vi "FRCts20_Backend_Processor.vi"() -> ()   [LabVIEW 2014, in "FRCts20_Backend_Engine.lvlib"]
doc: "The Processor VI represents the CPU for the Web Service system. All command messages are routed and handled by the central processor"
uses:
  FRCts20_Backend_Engine.lvlib
  FRCts20_Backend_FGVOperation.ctl
  FRCts20_Backend_DequeueDataOperations.ctl
  Dependencies/AMC/_SubVIs/TypeDefs/Message.ctl
  Dependencies/Keyed Array/KeyedArray.ctl
  <vilib>/addons/database/Connection.llb/DB Tools Open Connec (String).vi
  Dependencies/AMC/AMC.lvlib
  <vilib>/addons/database/NI_Database_API.lvlib
  INI_Accessor/FRCts20_Backend_INI Controller.lvclass
  Dependencies/Keyed Array/Tools_KeyedArray.lvlib
panel:
  out "Status":string
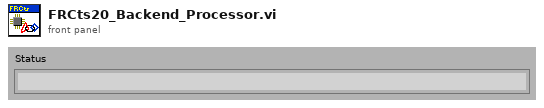
[diagram p1: front panel]
types:
  T1 = typedef "FRCts20_Backend_Engine.lvlib/FRCts20_Backend_EngineRefnums.ctl" = cluster{"Message Queue Methods":T2, "Message Queue Returns":T2, "Data Store Path":path, "Database Refnum":T3, "INI":refnum<class "FRCts20_Backend_INI Controller.lvclass">}
  T2 = typedef "AMC.lvlib/Message Queue.ctl" = refnum<queue>
  T3 = typedef "NI_Database_API.lvlib/Conn ObjectReference.ctl" = refnum<k1>
  T4 = typedef "FRCts20_Backend_Engine.lvlib/FRCts20_Backend_DequeueDataOperations.ctl" = enum16{"Initialize", "DequeueDataReturn", "GetQueues"}
  T5 = typedef "FRCts20_Backend_Engine.lvlib/FRCts20_Backend_FGVOperation.ctl" = enum16{"Initialize", "EnqueueMessage", "EnqueueDataReturn", "FlushMessage", "FlushDataReturn"}
  T6 = typedef "AMC.lvlib/Message.ctl" = cluster{"Name":string, "Value":string, "Attributes":T7, "Receiver Host":string, "Receiver Process":string, "Source Host":string, "Source Process":string, "Priority Message":bool, "Acknowledge Message":bool}
  T7 = typedef "Tools_KeyedArray.lvlib/KeyedArray.ctl" = cluster{"keys":string[], "values":string[]}
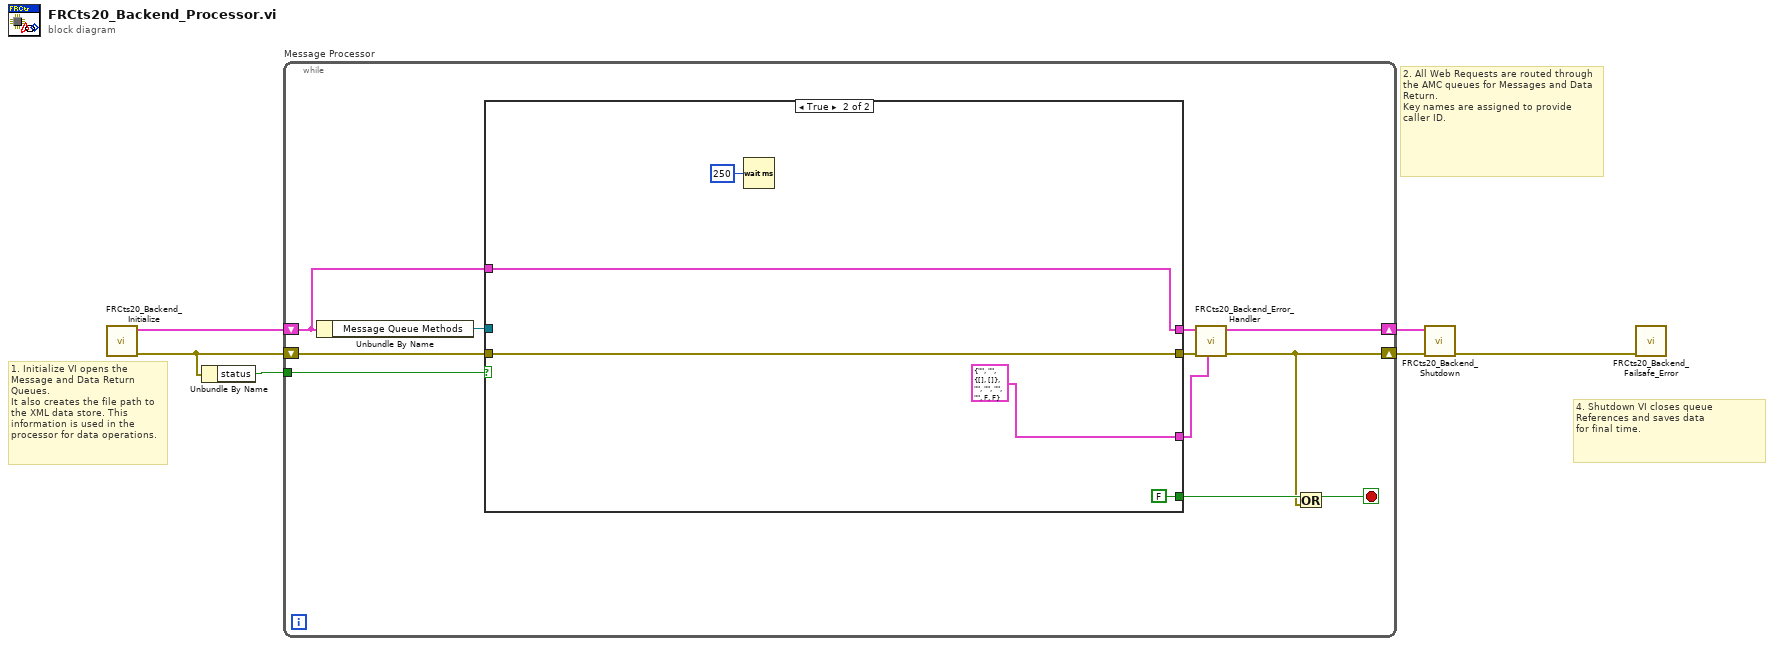
[diagram p0: block diagram]
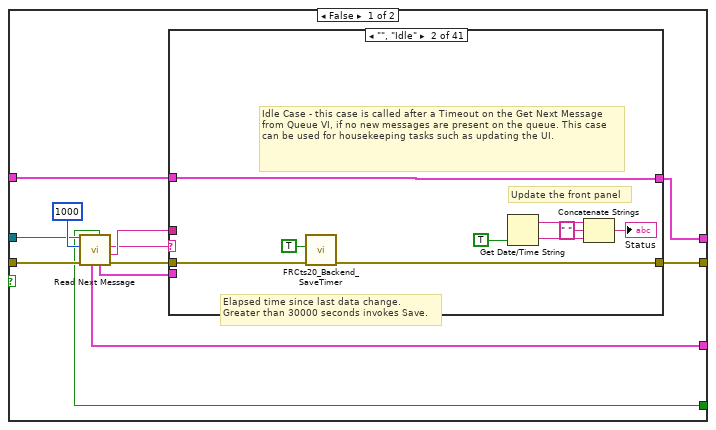
[diagram p2: hidden frame]
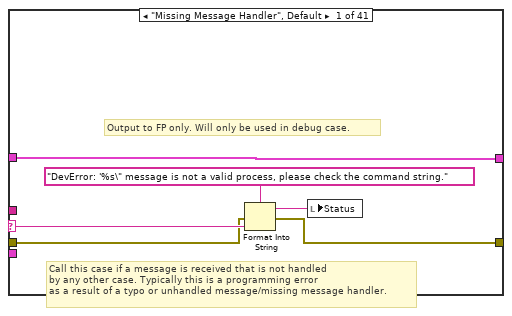
[diagram p3: hidden frame]
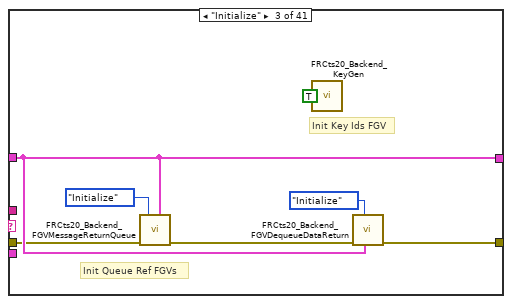
[diagram p4: hidden frame]
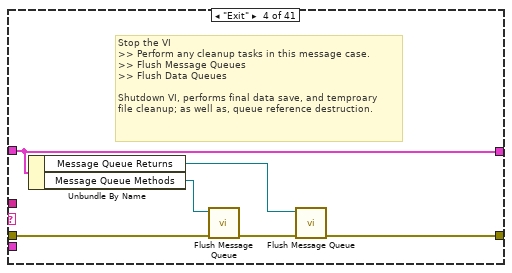
[diagram p5: hidden frame]
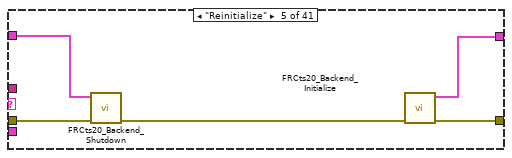
[diagram p6: hidden frame]
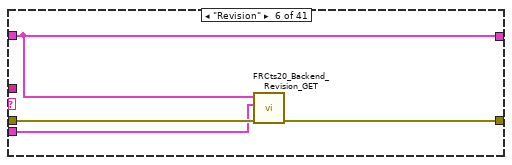
[diagram p7: hidden frame]
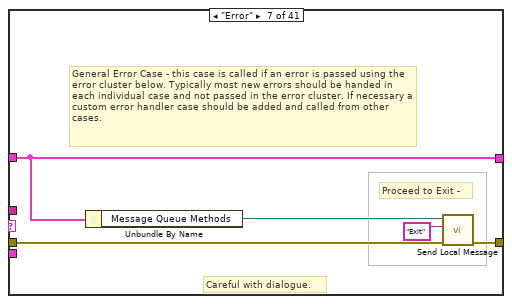
[diagram p8: hidden frame]
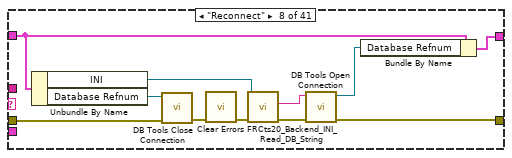
[diagram p9: hidden frame]
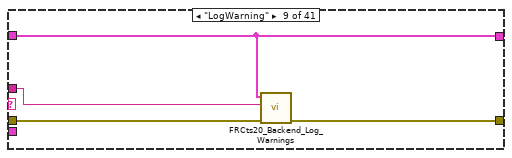
[diagram p10: hidden frame]
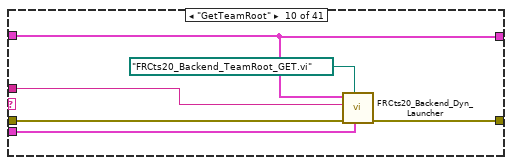
[diagram p11: hidden frame]
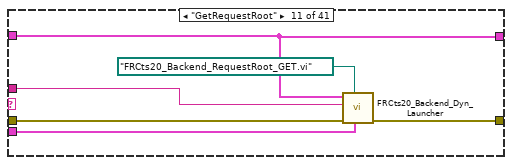
[diagram p12: hidden frame]
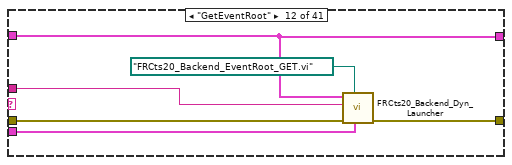
[diagram p13: hidden frame]
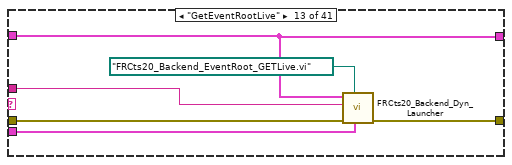
[diagram p14: hidden frame]
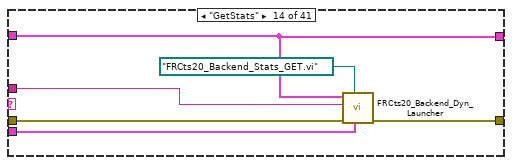
[diagram p15: hidden frame]
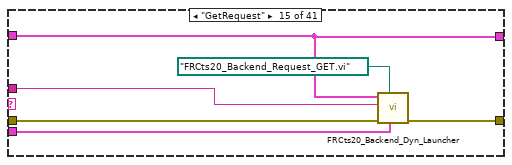
[diagram p16: hidden frame]
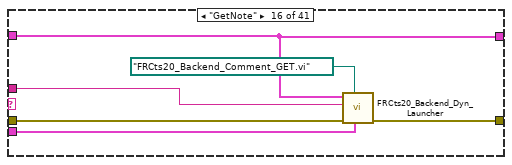
[diagram p17: hidden frame]
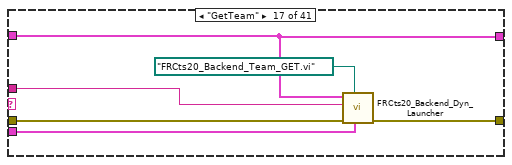
[diagram p18: hidden frame]
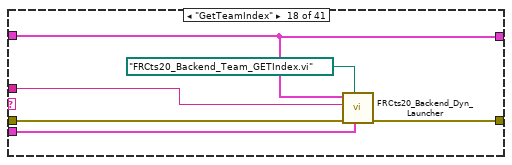
[diagram p19: hidden frame]
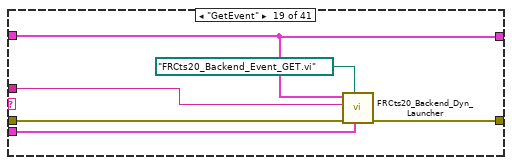
[diagram p20: hidden frame]
diagram:
  # "2. All Web Requests are routed through\nthe AMC queues for Messages and Data Return.\nKey names are assigned to provide caller ID."
  # "4. Shutdown VI closes queue References and saves data\nfor final time."
  # "1. Initialize VI opens the Message and Data Return Queues.\nIt also creates the file path to the XML data store. This \ninformation is used in the processor for data operations."
  n1 = call "FRCts20_Backend_Initialize.vi"() -> ("error out"=w2:errorcluster, "Engine_Refnums"=w5:T1)  [unwired: 10 in]
  n2 = Unbundle By Name(w2) -> ("status"=w1:bool)
  n3 = while "Message Processor" {
    shift-left: w2 -> [w10]
    shift-right: [w7] -> w6
    shift-right: [w12] -> w3
    shift-left: w5 -> [w16]
    tunnel: w1 -> [w11]
    stop <- w8 stop-if-true
    n4 = Unbundle By Name(w16) -> ("Message Queue Methods"=w17:T2)
    n5 = case shown="True" w11 {
      tunnel: w17 -> [w27 _]
      tunnel: w16 -> [w24 w290]
      tunnel: [w22 T6 {"Name"="", "Value"="", "Attributes"={"keys"=[], "values"=[]}, "Receiver Host"="", "Receiver Process"="", "Source Host"="", "Source Process"="", "Priority Message"=FALSE, "Acknowledge Message"=FALSE} ("Message")] -> w15
      tunnel: [w21 w288] -> w14
      tunnel: [w20 w290] -> w13
      tunnel: w10 -> [w19 w288]
      tunnel: [w18 FALSE ("Exit Process")] -> w9
      frame False {
        n6 = call "Read Next Message.vi"("error in (no error)"=w19, "timeout (1ms)"=1000 ("Timeout"), "Message Queue in"=w27) -> ("error out"=w29:errorcluster, "Message Value"=w26:string, "Message Name"=w23:string, "Message Attributes"=w25:T7, "Exit Process"=w18:bool, "Message"=w22:T6)  [unwired: 2 in, 1 out]
        n7 = case shown="\"\", \"Idle\"" w23 {
          selector: w23 -> [w35 _ _ _ _ _ _ _ _ _ _ _ _ _ _ _ _ _ _ _ _ _ _ _ _ _ _ _ _ _ _ _ _ _ _ _ _ _ _ _ _]
          tunnel: w29 -> [w31 w38 w46 w57 w61 w66 w68 w81 w85 w90 w96 w102 w108 w114 w120 w126 w132 w138 w144 w150 w156 w162 w168 w174 w180 w186 w192 w198 w204 w210 w216 w222 w228 w234 w240 w246 w252 w258 w264 w270 w277]
          tunnel: w26 -> [_ _ _ _ _ _ _ _ w83 w89 w95 w101 w107 w113 w119 w125 w131 w137 w143 w149 w155 w161 w167 w173 w179 w185 w191 w197 w203 w209 w215 w221 w227 w233 w239 w245 w251 w257 w263 w269 w276]
          tunnel: w25 -> [_ _ _ _ _ w63 _ _ _ w91 w97 w103 w109 w115 w121 w127 w133 w139 w145 w151 w157 w163 w169 w175 w181 w187 w193 w199 w205 w211 w217 w223 w229 w235 w241 w247 w253 w259 w265 w271 w278]
          tunnel: w24 -> [w33 w39 w47 w53 w60 w64 w67 w76 w86 w92 w98 w104 w110 w116 w122 w128 w134 w140 w146 w152 w158 w164 w170 w176 w182 w188 w194 w200 w206 w212 w218 w224 w230 w236 w242 w248 w254 w260 w266 w272 w273]
          tunnel: [w33 w39 w47 w53 w58 w64 w67 w77 w86 w92 w98 w104 w110 w116 w122 w128 w134 w140 w146 w152 w158 w164 w170 w176 w182 w188 w194 w200 w206 w212 w218 w224 w230 w236 w242 w248 w254 w260 w266 w272 w273] -> w20
          tunnel: [w30 w36 w45 w52 w59 w65 w69 w73 w84 w87 w93 w99 w105 w111 w117 w123 w129 w135 w141 w147 w153 w159 w165 w171 w177 w183 w189 w195 w201 w207 w213 w219 w225 w231 w237 w243 w249 w255 w261 w267 w274] -> w21
          frame "Missing Message Handler", Default {
            # "Output to FP only. Will only be used in debug case."
            # "Call this case if a message is received that is not handled \nby any other case. Typically this is a programming error\nas a result of a typo or unhandled message/missing message handler."
            n8 = Format Into String(format string="DevError: '%s\" message is not a valid process, please check the command string." ("message"), error in=w31, w35) -> (resulting string=w32:string, error out=w30:errorcluster)  [unwired: 1 in]
            n9 = local write "Status"(w32) -> ()
          }
          frame "", "Idle" {
            # "Elapsed time since last data change. \nGreater than 30000 seconds invokes Save."
            # "Update the front panel"
            # "Idle Case - this case is called after a Timeout on the Get Next Message from Queue VI, if no new messages are present on the queue. This case can be used for housekeeping tasks such as updating the UI."
            n10 = call "FRCts20_Backend_SaveTimer.vi"("error in (no error)"=w38, "Data Changed?"=TRUE) -> ("error out"=w36:errorcluster)  [unwired: 9 in]
            n11 = Get Date/Time String(want seconds? (F)=TRUE) -> (date string=w44:string, time string=w43:string)  [unwired: 2 out]
            n12 = Concatenate Strings(w44, " " ("string"), w43) -> (→"Status":string)
          }
          frame "Initialize" {
            # "Initialize competition start\ndate for stats generation"
            # "Init Queue Ref FGVs"
            # "Init Key Ids FGV"
            # "Primary Reference Initialization for Send/Return Queues"
            n13 = call "FRCts20_Backend_FGVMessageReturnQueue.vi"("Engine_Refnums"=w47, "Operation"=FRCts20_Backend_FGVOperation."Initialize", "error in (no error)"=w46) -> ("error out"=w50:errorcluster)  [unwired: 7 in, 1 out]
            n14 = call "FRCts20_Backend_KeyGen.vi"("Init?"=TRUE) -> ()  [unwired: 26 in, 1 out]
            n15 = call "FRCts20_Backend_FGVDequeueDataReturn.vi"("Engine_Refnums"=w47, "Operation"=FRCts20_Backend_DequeueDataOperations."Initialize", "error in (no error)"=w50) -> ("error out"=w45:errorcluster)  [unwired: 4 in, 4 out]
          }
          frame "Exit" {
            # "Stop the VI\n>> Perform any cleanup tasks in this message case.\n>> Flush Message Queues\n>> Flush Data Queues\n\nShutdown VI, performs final data save, and temproary\nfile cleanup; as well as, queue reference destruction."
            n16 = Unbundle By Name(w53) -> ("Message Queue Returns"=w54:T2, "Message Queue Methods"=w55:T2)
            n17 = call "Flush Message Queue.vi"("error in (no error)"=w57, "Message Queue in"=w55) -> ("error out"=w56:errorcluster)  [unwired: 7 in, 1 out]
            n18 = call "Flush Message Queue.vi"("error in (no error)"=w56, "Message Queue in"=w54) -> ("error out"=w52:errorcluster)  [unwired: 7 in, 1 out]
          }
          frame "Reinitialize" {
            n19 = call "FRCts20_Backend_Shutdown.vi"("error in (no error)"=w61, "Engine_Refnums"=w60) -> ("error out"=w62:errorcluster)  [unwired: 9 in]
            n20 = call "FRCts20_Backend_Initialize.vi"("error in (no error)"=w62) -> ("error out"=w59:errorcluster, "Engine_Refnums"=w58:T1)  [unwired: 9 in]
          }
          frame "Revision" {
            n21 = call "FRCts20_Backend_Revision_GET.vi"("error in (no error)"=w66, "Message Attributes"=w63, "Engine_Refnums"=w64) -> ("error out"=w65:errorcluster)  [unwired: 8 in]
          }
          frame "Error" {
            (unwired) errorcluster {"status"=FALSE, "code"=0, "source"=""} ("error out")
            # "Careful with dialogue."
            # "Proceed to Exit -"
            # "General Error Case - this case is called if an error is passed using the error cluster below. Typically most new errors should be handed in each individual case and not passed in the error cluster. If necessary a custom error handler case should be added and called from other cases."
            n22 = Unbundle By Name(w67) -> ("Message Queue Methods"=w70:T2)
            n23 = call "Send Local Message.vi"("error in (no error)"=w68, "Message Name"="Exit", "Message Queue in"=w70) -> ("error out"=w69:errorcluster)  [unwired: 3 in, 5 out]
          }
          frame "Reconnect" {
            n24 = Unbundle By Name(w76) -> ("INI"=w78:refnum<class "FRCts20_Backend_INI Controller.lvclass">, "Database Refnum"=w82:T3)
            n25 = call <vilib>:"DB Tools Close Connection.vi"("error in (no error)"=w81, "connection reference"=w82) -> ("error out"=w80:errorcluster)  [unwired: 5 in]
            n26 = call <vilib>:"Clear Errors.vi"("error in (no error)"=w80) -> ("error out"=w79:errorcluster)  [unwired: 5 in, 1 out]
            n27 = call "FRCts20_Backend_INI_Read_DB_String.vi"("error in (no error)"=w79, "INI Controller in"=w78) -> ("error out"=w74:errorcluster, "Connection String"=w75:string)  [unwired: 7 in, 1 out]
            n28 = call-poly <vilib>:"DB Tools Open Connection.vi"("error in (no error)"=w74, "connection information"=w75) -> ("error out"=w73:errorcluster, "connection reference"=w72:T3)  [unwired: 6 in]
            n29 = Bundle By Name(cluster=w76, "Database Refnum"=w72) -> (w77:T1)
          }
          frame "LogWarning" {
            n30 = call "FRCts20_Backend_Log_Warnings.vi"("error in (no error)"=w85, "Data"=w83, "Engine_Refnums"=w86) -> ("error out"=w84:errorcluster)  [unwired: 8 in]
          }
          frame "GetTeamRoot" {
            n31 = call "FRCts20_Backend_Dyn_Launcher.vi"("Message Attributes"=w91, "VI Name"=path "FRCts20_Backend_TeamRoot_GET.vi" ("VI Path"), "error in (no error)"=w90, "Data"=w89, "Engine_Refnums"=w92) -> ("error out"=w87:errorcluster)  [unwired: 6 in]
          }
          frame "GetRequestRoot" {
            n32 = call "FRCts20_Backend_Dyn_Launcher.vi"("Message Attributes"=w97, "VI Name"=path "FRCts20_Backend_RequestRoot_GET.vi" ("VI Path"), "error in (no error)"=w96, "Data"=w95, "Engine_Refnums"=w98) -> ("error out"=w93:errorcluster)  [unwired: 6 in]
          }
          frame "GetEventRoot" {
            n33 = call "FRCts20_Backend_Dyn_Launcher.vi"("Message Attributes"=w103, "VI Name"=path "FRCts20_Backend_EventRoot_GET.vi" ("VI Path"), "error in (no error)"=w102, "Data"=w101, "Engine_Refnums"=w104) -> ("error out"=w99:errorcluster)  [unwired: 6 in]
          }
          frame "GetEventRootLive" {
            n34 = call "FRCts20_Backend_Dyn_Launcher.vi"("Message Attributes"=w109, "VI Name"=path "FRCts20_Backend_EventRoot_GETLive.vi" ("VI Path"), "error in (no error)"=w108, "Data"=w107, "Engine_Refnums"=w110) -> ("error out"=w105:errorcluster)  [unwired: 6 in]
          }
          frame "GetStats" {
            n35 = call "FRCts20_Backend_Dyn_Launcher.vi"("Message Attributes"=w115, "VI Name"=path "FRCts20_Backend_Stats_GET.vi" ("VI Path"), "error in (no error)"=w114, "Data"=w113, "Engine_Refnums"=w116) -> ("error out"=w111:errorcluster)  [unwired: 6 in]
          }
          frame "GetRequest" {
            n36 = call "FRCts20_Backend_Dyn_Launcher.vi"("Message Attributes"=w121, "VI Name"=path "FRCts20_Backend_Request_GET.vi" ("VI Path"), "error in (no error)"=w120, "Data"=w119, "Engine_Refnums"=w122) -> ("error out"=w117:errorcluster)  [unwired: 6 in]
          }
          frame "GetNote" {
            n37 = call "FRCts20_Backend_Dyn_Launcher.vi"("Message Attributes"=w127, "VI Name"=path "FRCts20_Backend_Comment_GET.vi" ("VI Path"), "error in (no error)"=w126, "Data"=w125, "Engine_Refnums"=w128) -> ("error out"=w123:errorcluster)  [unwired: 6 in]
          }
          frame "GetTeam" {
            n38 = call "FRCts20_Backend_Dyn_Launcher.vi"("Message Attributes"=w133, "VI Name"=path "FRCts20_Backend_Team_GET.vi" ("VI Path"), "error in (no error)"=w132, "Data"=w131, "Engine_Refnums"=w134) -> ("error out"=w129:errorcluster)  [unwired: 6 in]
          }
          frame "GetTeamIndex" {
            n39 = call "FRCts20_Backend_Dyn_Launcher.vi"("Message Attributes"=w139, "VI Name"=path "FRCts20_Backend_Team_GETIndex.vi" ("VI Path"), "error in (no error)"=w138, "Data"=w137, "Engine_Refnums"=w140) -> ("error out"=w135:errorcluster)  [unwired: 6 in]
          }
          frame "GetEvent" {
            n40 = call "FRCts20_Backend_Dyn_Launcher.vi"("Message Attributes"=w145, "VI Name"=path "FRCts20_Backend_Event_GET.vi" ("VI Path"), "error in (no error)"=w144, "Data"=w143, "Engine_Refnums"=w146) -> ("error out"=w141:errorcluster)  [unwired: 6 in]
          }
          frame "GetEventFiltered" {
            n41 = call "FRCts20_Backend_Dyn_Launcher.vi"("Message Attributes"=w151, "VI Name"=path "FRCts20_Backend_Event_GETFiltered.vi" ("VI Path"), "error in (no error)"=w150, "Data"=w149, "Engine_Refnums"=w152) -> ("error out"=w147:errorcluster)  [unwired: 6 in]
          }
          frame "GetDivision" {
            n42 = call "FRCts20_Backend_Dyn_Launcher.vi"("Message Attributes"=w157, "VI Name"=path "FRCts20_Backend_Division_GET.vi" ("VI Path"), "error in (no error)"=w156, "Data"=w155, "Engine_Refnums"=w158) -> ("error out"=w153:errorcluster)  [unwired: 6 in]
          }
          frame "PostRequestRoot" {
            n43 = call "FRCts20_Backend_Dyn_Launcher.vi"("Message Attributes"=w163, "VI Name"=path "FRCts20_Backend_RequestRoot_POST.vi" ("VI Path"), "error in (no error)"=w162, "Data"=w161, "Engine_Refnums"=w164) -> ("error out"=w159:errorcluster)  [unwired: 6 in]
          }
          frame "PostNote" {
            n44 = call "FRCts20_Backend_Dyn_Launcher.vi"("Message Attributes"=w169, "VI Name"=path "FRCts20_Backend_Comment_POST.vi" ("VI Path"), "error in (no error)"=w168, "Data"=w167, "Engine_Refnums"=w170) -> ("error out"=w165:errorcluster)  [unwired: 6 in]
          }
          frame "PostEventRoot" {
            n45 = call "FRCts20_Backend_Dyn_Launcher.vi"("Message Attributes"=w175, "VI Name"=path "FRCts20_Backend_EventRoot_POST.vi" ("VI Path"), "error in (no error)"=w174, "Data"=w173, "Engine_Refnums"=w176) -> ("error out"=w171:errorcluster)  [unwired: 6 in]
          }
          frame "PostDivision" {
            n46 = call "FRCts20_Backend_Dyn_Launcher.vi"("Message Attributes"=w181, "VI Name"=path "FRCts20_Backend_Division_POST.vi" ("VI Path"), "error in (no error)"=w180, "Data"=w179, "Engine_Refnums"=w182) -> ("error out"=w177:errorcluster)  [unwired: 6 in]
          }
          frame "PostTeamRoot" {
            n47 = call "FRCts20_Backend_Dyn_Launcher.vi"("Message Attributes"=w187, "VI Name"=path "FRCts20_Backend_TeamRoot_POST.vi" ("VI Path"), "error in (no error)"=w186, "Data"=w185, "Engine_Refnums"=w188) -> ("error out"=w183:errorcluster)  [unwired: 6 in]
          }
          frame "PutRequest" {
            n48 = call "FRCts20_Backend_Dyn_Launcher.vi"("Message Attributes"=w193, "VI Name"=path "FRCts20_Backend_Request_PUT.vi" ("VI Path"), "error in (no error)"=w192, "Data"=w191, "Engine_Refnums"=w194) -> ("error out"=w189:errorcluster)  [unwired: 6 in]
          }
          frame "PutEvent" {
            n49 = call "FRCts20_Backend_Dyn_Launcher.vi"("Message Attributes"=w199, "VI Name"=path "FRCts20_Backend_Event_PUT.vi" ("VI Path"), "error in (no error)"=w198, "Data"=w197, "Engine_Refnums"=w200) -> ("error out"=w195:errorcluster)  [unwired: 6 in]
          }
          frame "PutDivision" {
            n50 = call "FRCts20_Backend_Dyn_Launcher.vi"("Message Attributes"=w205, "VI Name"=path "FRCts20_Backend_Division_PUT.vi" ("VI Path"), "error in (no error)"=w204, "Data"=w203, "Engine_Refnums"=w206) -> ("error out"=w201:errorcluster)  [unwired: 6 in]
          }
          frame "PutDeleteDivision" {
            n51 = call "FRCts20_Backend_Dyn_Launcher.vi"("Message Attributes"=w211, "VI Name"=path "FRCts20_Backend_Division_PUT_DELETE.vi" ("VI Path"), "error in (no error)"=w210, "Data"=w209, "Engine_Refnums"=w212) -> ("error out"=w207:errorcluster)  [unwired: 6 in]
          }
          frame "PutTeam" {
            n52 = call "FRCts20_Backend_Dyn_Launcher.vi"("Message Attributes"=w217, "VI Name"=path "FRCts20_Backend_Team_PUT.vi" ("VI Path"), "error in (no error)"=w216, "Data"=w215, "Engine_Refnums"=w218) -> ("error out"=w213:errorcluster)  [unwired: 6 in]
          }
          frame "PutNote" {
            n53 = call "FRCts20_Backend_Dyn_Launcher.vi"("Message Attributes"=w223, "VI Name"=path "FRCts20_Backend_Comment_PUT.vi" ("VI Path"), "error in (no error)"=w222, "Data"=w221, "Engine_Refnums"=w224) -> ("error out"=w219:errorcluster)  [unwired: 6 in]
          }
          frame "DeleteRequest" {
            n54 = call "FRCts20_Backend_Dyn_Launcher.vi"("Message Attributes"=w229, "VI Name"=path "FRCts20_Backend_Request_DELETE.vi" ("VI Path"), "error in (no error)"=w228, "Data"=w227, "Engine_Refnums"=w230) -> ("error out"=w225:errorcluster)  [unwired: 6 in]
          }
          frame "DeleteNote" {
            n55 = call "FRCts20_Backend_Dyn_Launcher.vi"("Message Attributes"=w235, "VI Name"=path "FRCts20_Backend_Comment_DELETE.vi" ("VI Path"), "error in (no error)"=w234, "Data"=w233, "Engine_Refnums"=w236) -> ("error out"=w231:errorcluster)  [unwired: 6 in]
          }
          frame "DeleteDivision" {
            n56 = call "FRCts20_Backend_Dyn_Launcher.vi"("Message Attributes"=w241, "VI Name"=path "FRCts20_Backend_Division_DELETE.vi" ("VI Path"), "error in (no error)"=w240, "Data"=w239, "Engine_Refnums"=w242) -> ("error out"=w237:errorcluster)  [unwired: 6 in]
          }
          frame "DeleteEvent" {
            n57 = call "FRCts20_Backend_Dyn_Launcher.vi"("Message Attributes"=w247, "VI Name"=path "FRCts20_Backend_Event_DELETE.vi" ("VI Path"), "error in (no error)"=w246, "Data"=w245, "Engine_Refnums"=w248) -> ("error out"=w243:errorcluster)  [unwired: 6 in]
          }
          frame "DeleteTeam" {
            n58 = call "FRCts20_Backend_Dyn_Launcher.vi"("Message Attributes"=w253, "VI Name"=path "FRCts20_Backend_Team_DELETE.vi" ("VI Path"), "error in (no error)"=w252, "Data"=w251, "Engine_Refnums"=w254) -> ("error out"=w249:errorcluster)  [unwired: 6 in]
          }
          frame "SNSPublish" {
            n59 = call "FRCts20_Backend_Dyn_Launcher.vi"("Message Attributes"=w259, "VI Name"=path "FRCts20_Backend_SNS_Publish.vi" ("VI Path"), "error in (no error)"=w258, "Data"=w257, "Engine_Refnums"=w260) -> ("error out"=w255:errorcluster)  [unwired: 6 in]
          }
          frame "SNSSubscribe" {
            n60 = call "FRCts20_Backend_Dyn_Launcher.vi"("Message Attributes"=w265, "VI Name"=path "FRCts20_Backend_SNS_Subscribe.vi" ("VI Path"), "error in (no error)"=w264, "Data"=w263, "Engine_Refnums"=w266) -> ("error out"=w261:errorcluster)  [unwired: 6 in]
          }
          frame "GetClosedRequests" {
            n61 = call "FRCts20_Backend_Dyn_Launcher.vi"("Message Attributes"=w271, "VI Name"=path "FRCts20_Backend_ClosedRequests.vi" ("VI Path"), "error in (no error)"=w270, "Data"=w269, "Engine_Refnums"=w272) -> ("error out"=w267:errorcluster)  [unwired: 6 in]
          }
          frame "SaveXMLData" {
            n62 = disable-structure shown="Disabled" {
              disable-tunnel: w273 -> [w284 _]
              disable-tunnel: w278 -> [w283 _]
              disable-tunnel: w277 -> [w282 w285]
              disable-tunnel: w276 -> [w281 _]
              disable-tunnel: [w279 w285] -> w275
              frame Disabled {
                n63 = call "FRCts20_Backend_Dyn_Launcher.vi"("Message Attributes"=w283, "VI Name"=path "FRCts20_Backend_SaveXMLData.vi" ("VI Path"), "error in (no error)"=w282, "Data"=w281, "Engine_Refnums"=w284) -> ("error out"=w279:errorcluster)  [unwired: 6 in]
              }
              frame Enabled {
              }
            }
            n64 = call "FRCts20_Backend_Ping_DB.vi"("error in (no error)"=w275, "Engine_Refnums"=w273) -> ("error out"=w274:errorcluster)  [unwired: 9 in]
          }
        }
      }
      frame True {
        n65 = Wait (ms)(milliseconds to wait=u32 250) -> ()  [unwired: 1 out]
      }
    }
    n66 = call "FRCts20_Backend_Error_Handler.vi"("Failed Message"=w15, "Error In"=w14, "Engine_Refnums In"=w13) -> ("error out"=w7:errorcluster, "Engine_Refnums Out"=w12:T1)  [unwired: 7 in]
    n67 = Or(x=w9, y=w7) -> (x .or. y?=w8:bool)
  }
  n68 = call "FRCts20_Backend_Shutdown.vi"("error in (no error)"=w6, "Engine_Refnums"=w3) -> ("error out"=w4:errorcluster)  [unwired: 9 in]
  n69 = call "FRCts20_Backend_Failsafe_Error.vi"("error in"=w4) -> ()  [unwired: 11 in]
